vi "splash.vi"() -> (0 "error out":errorcluster)   [LabVIEW 2019]
panel:
  out "element":picture
  in  "ok":bool
  # "Multi-PasS"
  # "ND\n\n\nmars 2025"
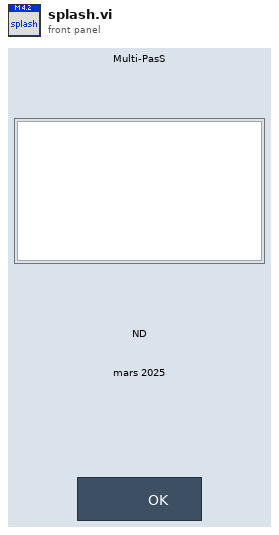
[diagram p1: front panel]
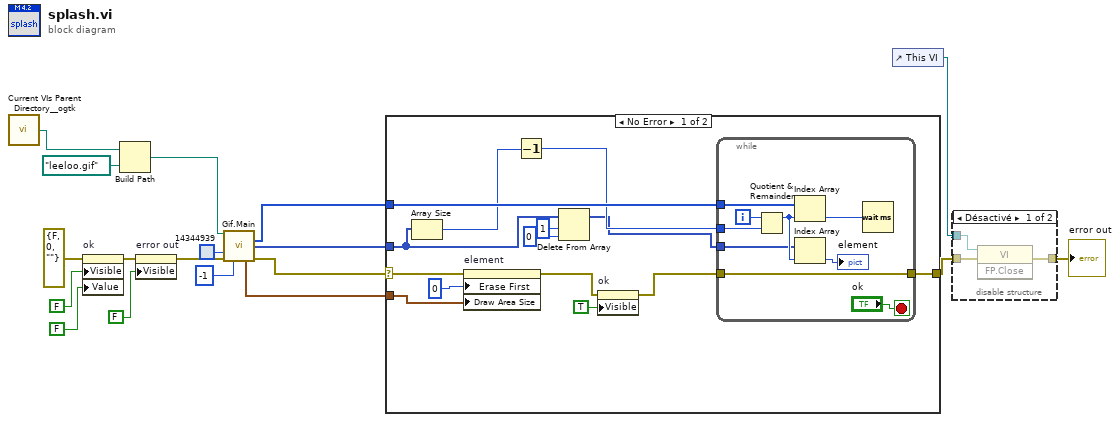
[diagram p0: block diagram]
diagram:
  n1 = call "Current VIs Parent Directory__ogtk.vi"() -> ("Parent Directory (+ Relative)"=w3:path)  [unwired: 5 in]
  n2 = property on="ok" class="Bool (strict)"(error in=errorcluster {"status"=FALSE, "code"=0, "source"=""} ("error in (no error)"), "Visible"=FALSE, "Value"=FALSE ("ok")) -> (error out=w13:errorcluster)  [unwired: 1 in, 1 out]
  n3 = Build Path(base path=w3, name or relative path=path "leeloo.gif") -> (appended path=w1:path)
  n4 = property on="error out" class="Clust (strict)"(error in=w13, "Visible"=FALSE) -> (error out=w6:errorcluster)  [unwired: 1 in, 1 out]
  n5 = call "Gif.Main.vi"("file path"=w1, "bgcolor"=u32 14344939, "error in (no error)"=w6, "image index"=-1) -> ("time"=w8:u32[], "images out"=w11:picture[], "image size"=w9:cluster{"Width":u32, "Height":u32}, "error out"=w10:errorcluster)  [unwired: 8 out]
  n6 = case shown="No Error" w10 {
    selector: w10 -> [w29 w42]
    tunnel: w8 -> [w31 _]
    tunnel: w9 -> [w28 _]
    tunnel: [w32 w42] -> w7
    tunnel: w11 -> [w22 _]
    frame No Error {
      n7 = Array Size(array=w22) -> (size(s)=w24:i32)
      n8 = property on="element" class="Pict"(error in=w29, "Erase First"=u8 0 ("Zuerst löschen"), "Draw Area Size"=w28) -> (error out=w27:errorcluster)  [unwired: 1 in, 1 out]
      n9 = Decrement(x=w24) -> (x-1=w23:i32)
      n10 = Delete From Array(array=w22, length=1 ("longueur"), index=0 ("indice")) -> (array with subset deleted=w19:picture[])  [unwired: 1 out]
      n11 = property on="ok" class="Bool (strict)"(error in=w27, "Visible"=TRUE) -> (error out=w26:errorcluster)  [unwired: 1 in, 1 out]
      n12 = while {
        tunnel: w31 -> [w36]
        tunnel: w26 -> [w38]
        tunnel: w23 -> [w40]
        tunnel: [w38] -> w32
        tunnel: w19 -> [w35]
        i -> [w41]
        stop <- "ok" stop-if-true
        n13 = Quotient & Remainder(x=w41, y=w40) -> (x-y*floor(x/y)=w39:i32)  [unwired: 1 out]
        n14 = Index Array(array=w36, index=w39) -> (element=w37:u32)
        n15 = Index Array(array=w35, index=w39) -> (element=→"element":picture)
        n16 = Wait (ms)(milliseconds to wait=w37) -> ()  [unwired: 1 out]
      }
    }
    frame Error {
    }
  }
  n17 = control-ref of="This VI"() -> (w18:refnum<vi>)
  n18 = disable-structure shown="Désactivé" {
    disable-tunnel: w18 -> [w45 _]
    disable-tunnel: [w44 _] -> w15
    disable-tunnel: w7 -> [w43 _]
    frame Disabled {
      n19 = invoke on="Invoke Node" class="VI" method="FP.Close"(reference=w45, error in=w43) -> (error out=w44:errorcluster)  [unwired: 1 in, 2 out]
    }
    frame Enabled {
    }
  }
  "error out" <- w15
